vi "Const text color.vi"() -> (2 "invalid num color":u32(colorbox)=9868950, 3 "valid num color":u32(colorbox))   [LabVIEW 2018, in "LF2R IDE.lvlib" / "LF2R IDE.lvclass"]
uses:
  LF2R IDE.lvclass
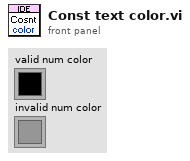
[diagram p1: front panel]
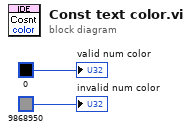
[diagram p0: block diagram]
diagram:
  "valid num color" <- u32 0 ("Color Box")
  "invalid num color" <- u32 9868950 ("Color Box 2")
